vi "Receive Query Response.vi"(0 "connection ID":refnum<k5>, 7 "Call Procedure?":bool, 9 "Timeout (60000ms)":i32=60000, 11 "error in (no error)":errorcluster) -> (4 "connection ID out":refnum<k5>, 6 "OK Packet Metadata":T2 {"Server Status" format="%.0x"}, 8 "Field Names":string[](array[string]), 10 "Return Data":string[][](array[string]), 15 "error out":errorcluster)   [LabVIEW 2014, in "hse-db.lvlib" / "MySQL (TCP).lvlib"]
uses:
  MySQL (TCP).lvlib
  Controls/OK Packet Metadata.ctl
  Controls/Return Packet Types.ctl
  Controls/Fields.ctl
  Controls/Character Set.ctl
  Controls/Data Types.ctl
panel:
  out "Array":T1[](array[typedef])
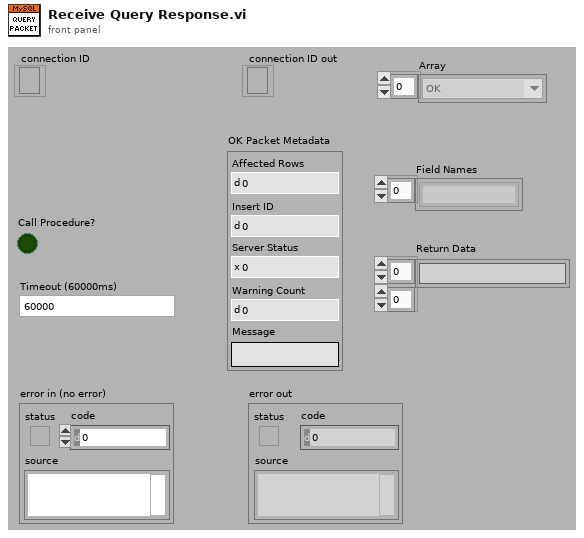
[diagram p1: front panel]
types:
  T1 = typedef "hse-db.lvlib/MySQL (TCP).lvlib/Return Packet Types.ctl" = enum16{"OK", "Result Set Header", "Error", "Field", "Row", "EOF"}
  T2 = typedef "hse-db.lvlib/MySQL (TCP).lvlib/OK Packet Metadata.ctl" = cluster{"Affected Rows":u64, "Insert ID":u64, "Server Status":u16, "Warning Count":u16, "Message":string}
  T3 = typedef "hse-db.lvlib/MySQL (TCP).lvlib/Fields.ctl" = cluster{"catalog":string, "schema":string, "table":string, "org_table":string, "name":string, "org_name":string, "next_length":u64, "character_set":T4, "column_length":u64, "column_type":T5, "flags":string, "decimals":string, "filler":string}
  T4 = typedef "hse-db.lvlib/MySQL (TCP).lvlib/Character Set.ctl" = enum16{"big5_chinese_ci", "dec8_swedish_ci", "cp850_general_ci", "hp8_english_ci", "koi8r_general_ci", "latin1_swedish_ci", "latin2_general_ci", "swe7_swedish_ci", "ascii_general_ci", "ujis_japanese_ci", "sjis_japanese_ci", "hebrew_general_ci", "tis620_thai_ci", "euckr_korean_ci", "koi8u_general_ci", "gb2312_chinese_ci", "greek_general_ci", "cp1250_general_ci", "gbk_chinese_ci", "latin5_turkish_ci", "armscii8_general_ci", "utf8_general_ci", "ucs2_general_ci", "cp866_general_ci", "keybcs2_general_ci", "macce_general_ci", "macroman_general_ci", "cp852_general_ci", "latin7_general_ci", "cp1251_general_ci", "utf16_general_ci", "utf16le_general_ci", "cp1256_general_ci", "cp1257_general_ci", "utf32_general_ci", "binary", "geostd8_general_ci", "cp932_japanese_ci", "eucjpms_japanese_ci", "gb18030_chinese_ci", "utf8mb4_0900_ai_ci"}
  T5 = typedef "hse-db.lvlib/MySQL (TCP).lvlib/Data Types.ctl" = enum16{"TINYINT", "SMALLINT", "MEDIUMINT", "INT", "BIGINT", "FLOAT", "DOUBLE", "NULL", "DECIMAL", "BIT", "CHAR", "VARCHAR", "TINYTEXT", "TEXT", "MEDIUMTEXT", "LONGTEXT", "BINARY", "VARBINARY", "TINYBLOB", "BLOB", "MEDIUMBLOB", "LONGBLOB", "ENUM", "SET", "DATE", "DATETIME", "TIME", "TIMESTAMP", "YEAR", "GEOMETRY"}
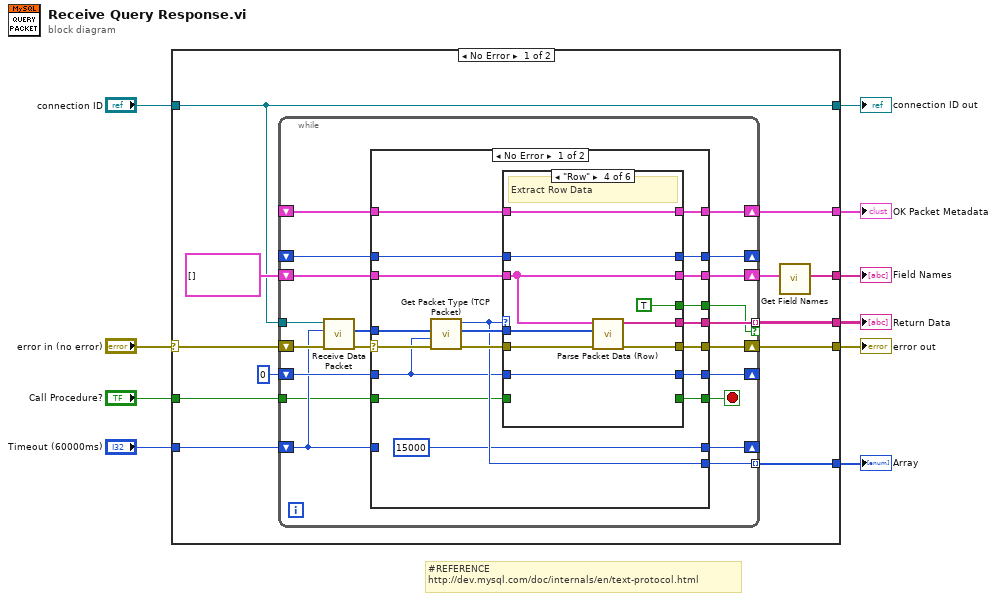
[diagram p0: block diagram]
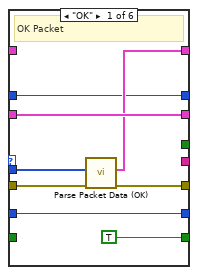
[diagram p2: hidden frame]
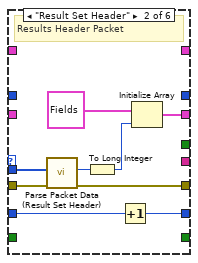
[diagram p3: hidden frame]
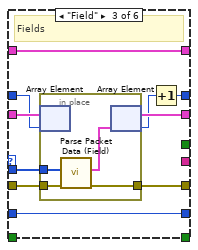
[diagram p4: hidden frame]
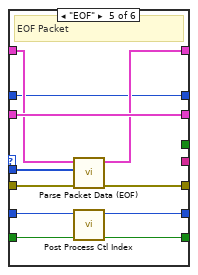
[diagram p5: hidden frame]
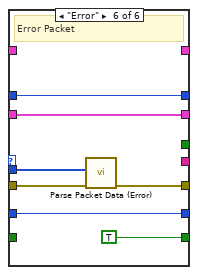
[diagram p6: hidden frame]
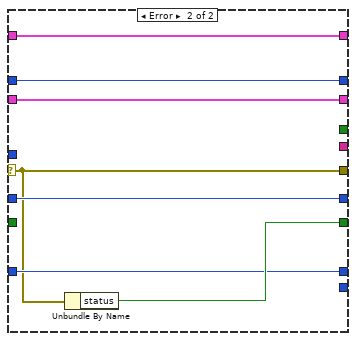
[diagram p7: hidden frame]
diagram:
  # "#REFERENCE\nhttp://dev.mysql.com/doc/internals/en/text-protocol.html"
  n1 = case shown="No Error" "error in (no error)" {
    selector: "error in (no error)" -> [w20 w128]
    tunnel: [w22 _] -> w8
    tunnel: [w21 w128] -> w10
    tunnel: "connection ID" -> [w11 w127]
    tunnel: [w11 w127] -> w6
    tunnel: "Timeout (60000ms)" -> [w17 _]
    tunnel: [w18 _] -> w4
    tunnel: [w15 _] -> w3
    tunnel: [w13 _] -> w2
    tunnel: "Call Procedure?" -> [w12 _]
    frame No Error {
      n2 = while {
        shift-right: [w41] -> w21
        shift-left: w20 -> [w40]
        shift-right: [w42] -> w22
        shift-left: _ -> [w37]
        shift-right: [w34] -> w19
        shift-left: T3[] [] -> [w35]
        shift-right: [w33] -> _
        shift-left: _ -> [w32]
        tunnel: [w31] -> w15 mode=indexing if=w30
        shift-right: [w29] -> _
        shift-left: u8 0 ("Counter out") -> [w28]
        tunnel: [w27] -> w13 mode=indexing
        shift-right: [w26] -> _
        shift-left: w17 -> [w25]
        tunnel: w12 -> [w24]
        tunnel: w11 -> [w23]
        stop <- w38 stop-if-true
        n3 = call "Receive Data Packet.vi"("error in"=w40, "Timeout (60000ms)"=w25, "connection ID"=w23) -> ("error out"=w36:errorcluster, "TCP/IP Data"=w39:u8[])  [unwired: 5 in, 2 out]
        n4 = case shown="No Error" w36 {
          selector: w36 -> [w55 w120]
          tunnel: [w61 w126] -> w42
          tunnel: [w60 w120] -> w41
          tunnel: w39 -> [w56 _]
          tunnel: [w43 w124] -> w38
          tunnel: w37 -> [w59 w126]
          tunnel: w35 -> [w58 w125]
          tunnel: [w57 w125] -> w34
          tunnel: [w52 w123] -> w33
          tunnel: w32 -> [w51 w123]
          tunnel: [w50 _] -> w31
          tunnel: [w49 _] -> w30
          tunnel: [w47 w121] -> w29
          tunnel: w28 -> [w46 w121]
          tunnel: [w48 _] -> w27
          tunnel: [15000 ("Timeout (60000ms)") w122] -> w26
          tunnel: w25 -> [_ w122]
          tunnel: w24 -> [w44 _]
          frame No Error {
            n5 = call "Get Packet Type (TCP Packet).vi"("Error In"=w55, "Ctl index"=w46, "TCP/IP Data in"=w56) -> ("Error Out"=w54:errorcluster, "TCP/IP Data out"=w53:u8[], "Return Packet Type"=w48:T1)  [unwired: 6 in]
            n6 = case shown="\"Row\"" w48 {
              tunnel: w53 -> [w68 w78 w87 w100 w109 w116]
              tunnel: [w65 _ w88 w101 w110 _] -> w61
              tunnel: w54 -> [w67 w77 w86 w99 w108 w119]
              tunnel: [w66 w76 w85 w98 w107 w118] -> w60
              tunnel: w59 -> [_ _ w88 w101 w111 _]
              tunnel: w58 -> [w69 _ w84 w93 w112 w117]
              tunnel: [w69 w74 w82 w93 w112 w117] -> w57
              tunnel: [w64 _ w80 w97 w106 w115] -> w52
              tunnel: w51 -> [w64 _ w83 w97 w106 w115]
              tunnel: [_ _ _ w96 _ _] -> w50
              tunnel: [_ _ _ TRUE _ _] -> w49
              tunnel: w46 -> [w63 w73 w79 w94 w105 w114]
              tunnel: [w63 w72 w79 w94 w104 w114] -> w47
              tunnel: w44 -> [_ _ _ _ w103 _]
              tunnel: [TRUE ("End") _ _ _ w102 TRUE ("End")] -> w43
              frame "OK" {
                # "OK Packet"
                n7 = call "Parse Packet Data (OK).vi"("Error In"=w67, "Recieved Bytes"=w68) -> ("Error Out"=w66:errorcluster, "Packet Metadata out"=w65:T2)  [unwired: 8 in]
              }
              frame "Result Set Header" {
                # "Results Header Packet"
                n8 = call "Parse Packet Data (Result Set Header).vi"("Error In"=w77, "Recieved Bytes"=w78) -> ("Error Out"=w76:errorcluster, "Field Count"=w71:u64)  [unwired: 8 in]
                n9 = To Long Integer(number=w71) -> (32bit integer=w70:i32)
                n10 = Increment(x=w73) -> (x+1=w72:u8)
                n11 = Initialize Array(T3 {"catalog"="", "schema"="", "table"="", "org_table"="", "name"="", "org_name"="", "next_length"=0, "character_set"=enum."big5_chinese_ci", "column_length"=0, "column_type"=enum."TINYINT", "flags"="", "decimals"="", "filler"=""} ("Fields"), w70) -> (w74:T3[])
              }
              frame "Field" {
                # "Fields"
                n12 = in-place {
                  in-place-border: w87 -> [w92]
                  in-place-border: w86 -> [w91]
                  in-place-border: [w90] -> w85
                  n13 = in-place-array #1(w84, w83) -> ()  [unwired: 1 out]
                  n14 = call "Parse Packet Data (Field).vi"("Error In"=w91, "Recieved Bytes"=w92) -> ("Error Out"=w90:errorcluster, "Fields"=w89:T3)  [unwired: 8 in]
                  n15 = in-place-array #1(w89) -> (w82:T3[], w81:i32)
                }
                n16 = Increment(x=w81) -> (x+1=w80:i32)
              }
              frame "Row" {
                # "Extract Row Data"
                n17 = call "Parse Packet Data (Row).vi"("Error In"=w99, "Recieved Bytes"=w100, "Fields"=w93) -> ("Error Out"=w98:errorcluster, "Row Data"=w96:string[])  [unwired: 6 in, 1 out]
              }
              frame "EOF" {
                # "EOF Packet"
                n18 = call "Parse Packet Data (EOF).vi"("Error In"=w108, "Recieved Bytes"=w109, "Packet Metadata In"=w111) -> ("Error Out"=w107:errorcluster, "Packet Metadata Out"=w110:T2)  [unwired: 7 in]
                n19 = call "Post Process Ctl Index.vi"("Call Procedure?"=w103, "Ctl Index in"=w105) -> ("Exit?"=w102:bool, "Ctl Index out"=w104:u8)  [unwired: 8 in]
              }
              frame "Error" {
                # "Error Packet"
                n20 = call "Parse Packet Data (Error).vi"("error in (no error)"=w119, "Recieved Bytes"=w116) -> ("error out"=w118:errorcluster)  [unwired: 9 in]
              }
            }
          }
          frame Error {
            n21 = Unbundle By Name(w120) -> ("status"=w124:bool)
          }
        }
      }
      n22 = call "Get Field Names.vi"("Fields"=w19) -> ("Field Names"=w18:string[])  [unwired: 10 in]
    }
    frame Error {
    }
  }
  "error out" <- w10
  "OK Packet Metadata" <- w8
  "Return Data" <- w3
  "connection ID out" <- w6
  "Field Names" <- w4
  "Array" <- w2
